vi "VISA.vi"(8 "에러 입력(에러 없음)":errorcluster, 10 "바이트 카운트":u32, 11 "VISA Configuration":T1 {"termination char\n(0xA = '\\n' = LF)" format="%.0x"; "flow control (0:none)" items=["None", "XON/XOFF", "RTS/CTS", "XON/XOFF & RTS/CTS", "DTR/DSR", "XON/XOFF & DTR/DSR"]; "stop bits (10: 1 bit)" items=["1.0"=10, "1.5"=15, "2.0"=20]; "data bits (8)" min=5 max=8 step=1}) -> (0 "에러 출력":errorcluster, 3 "read buffer":string)   [LabVIEW 2019]
uses:
  <vilib>/myRIO/Instrument Drivers/Onboard IO/UART/typedef/VISA Configuration.ctl
  <vilib>/Instr/_visa.llb/VISA Configure Serial Port (Instr).vi
  <vilib>/myRIO/Instrument Drivers/Onboard IO/UART/UART.lvlib
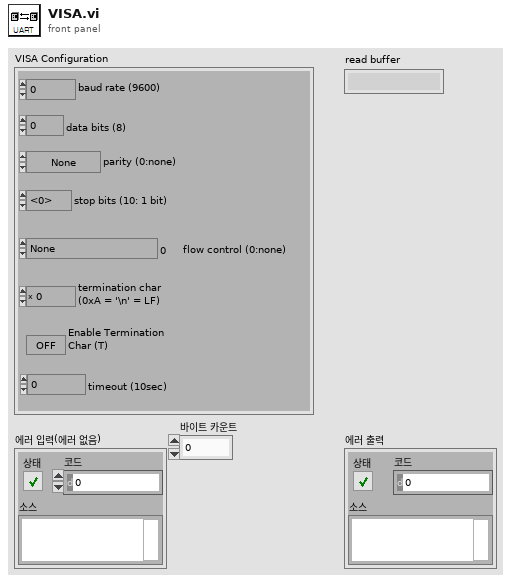
[diagram p1: front panel]
types:
  T1 = typedef "UART.lvlib/VISA Configuration.ctl" = cluster{"baud rate (9600)":u32, "data bits (8)":u16, "parity (0:none)":enum16{"None", "Odd", "Even", "Mark", "Space"}, "stop bits (10: 1 bit)":u16, "flow control (0:none)":u16, "termination char\n(0xA = '\\n' = LF) ":u8, "Enable Termination\nChar (T)":bool, "timeout (10sec)":u32}
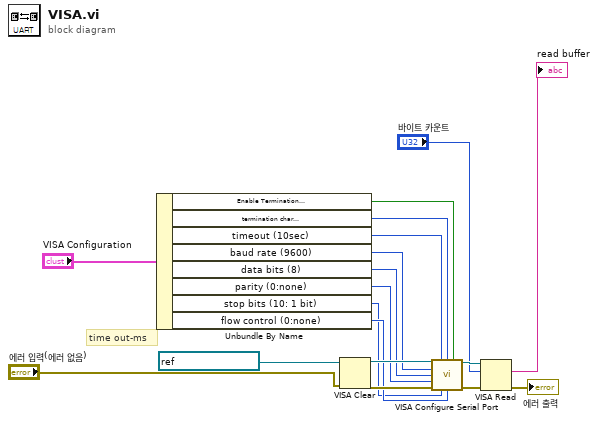
[diagram p0: block diagram]
diagram:
  # "time out-ms"
  n1 = Unbundle By Name("VISA Configuration") -> ("Enable Termination\nChar (T)"=w9:bool, "termination char\n(0xA = '\\n' = LF)"=w8:u8, "timeout (10sec)"=w7:u32, "baud rate (9600)"=w2:u32, "data bits (8)"=w3:u16, "parity (0:none)"=w4:enum16{"None", "Odd", "Even", "Mark", "Space"}, "stop bits (10: 1 bit)"=w5:u16, "flow control (0:none)"=w6:u16)
  n2 = VISA Clear(VISA resource name=refnum<visa-resource-name> "ASRL1::INSTR" ("VISA resource name in"), error in (no error)="에러 입력(에러 없음)") -> (VISA resource name out=w17:refnum<visa-resource-name>, error out=w15:errorcluster)
  n3 = call-poly "VISA Configure Serial Port"("VISA resource name"=w17, "timeout (10sec)"=w7, "termination char\n(0xA = '\\n' = LF)"=w8, "Enable Termination\nChar (T)"=w9, "baud rate (9600)"=w2, "data bits (8)"=w3, "parity (0:none)"=w4, "error in (no error)"=w15, "stop bits (10: 1 bit)"=w5, "flow control (0:none)"=w6) -> ("VISA resource name out"=w12:refnum<visa-resource-name>, "error out"=w11:errorcluster)  [unwired: 4 in]
  n4 = VISA Read(VISA resource name=w12, byte count="바이트 카운트", error in (no error)=w11) -> (read buffer=→"read buffer":string, error out=→"에러 출력":errorcluster)  [unwired: 2 out]
